vi "subSave_AcquireMC3DPhotoInfomation.vi"(7 "text":string="Z = 3481.00\rZou Lab\r2016/4/15 10:25:27\r============== \r============== \rCamera\rS/N: 003222\tLeft Cam\rnrow = \t2048\rncol = \t2048\rrow offset = \t0\rcol offset = \t0\rBinning =\t1\rExposure (msec) = \t200\r============== \rLight Ctrl and Global\rlaser\tDO\tAO(V)\r637    \t0\t0.00\r561    \t0\t0.00\r532    \t0\t0.00\r488    \t0\t0.00\r405    \t0\t0.00\rLED   \t0\t  --\rGlobal \t0\t  --\r============== \rTI-Ctrl\rObjective = \t6\t- empty 6 -\rCube Top = \t1\tCy5\rCube Bottom = \t1\t- empty 1 -\r============== \rStage Ctrl\rX Position = \t66.0000\rY Position = \t46.0000\r============== \rFilter Wheel\rFW Positon = \t1\r============== \r============== ", 8 "Total Num":i32, 9 "Crosswide":i32, 10 "Lengthwide":i32, 11 "Z value":string) -> (3 "text out":string)   [LabVIEW 2015]
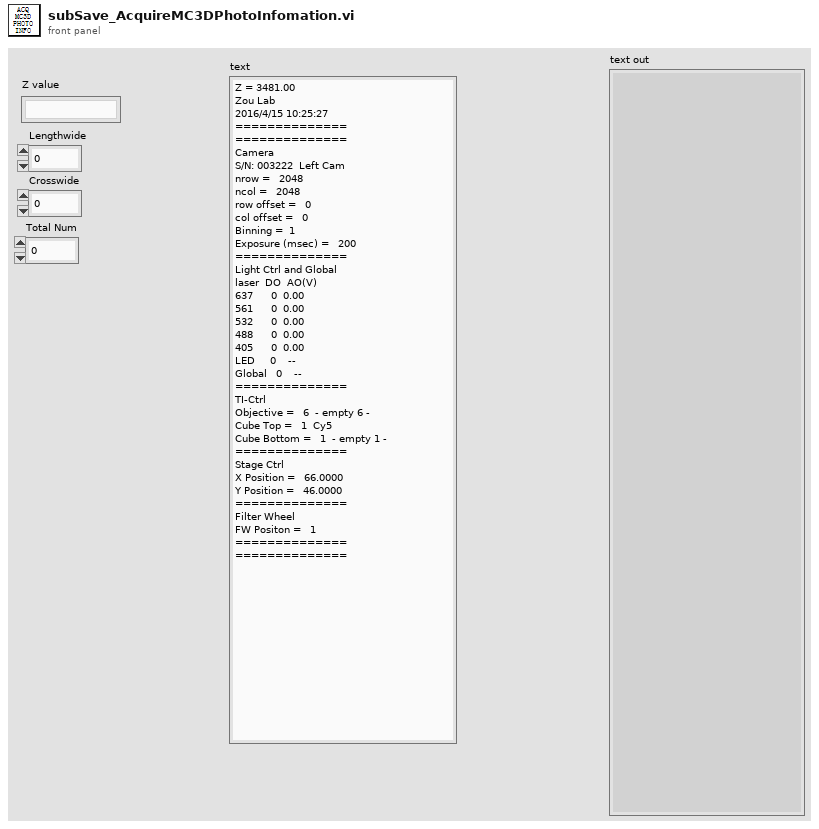
[diagram p1: front panel]
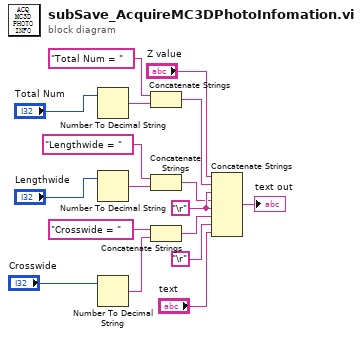
[diagram p0: block diagram]
diagram:
  w15 = "\r"
  n1 = Number To Decimal String(number="Total Num") -> (decimal integer string=w16:string)  [unwired: 1 in]
  n2 = Number To Decimal String(number="Lengthwide") -> (decimal integer string=w10:string)  [unwired: 1 in]
  n3 = Number To Decimal String(number="Crosswide") -> (decimal integer string=w6:string)  [unwired: 1 in]
  n4 = Concatenate Strings("Total Num = " ("string"), w16) -> (w17:string)
  n5 = Concatenate Strings("Lengthwide = " ("string"), w10) -> (w9:string)
  n6 = Concatenate Strings("Crosswide = " ("string"), w6) -> (w7:string)
  n7 = Concatenate Strings("Z value", w17, w15, w9, w15, w7, "\r", "text") -> (→"text out":string)
